vi "Set Velocity Setpoint.vi"(8 "error in (no error)":errorcluster, 10 "CCW Velocity (0 rad/s)":dbl, 11 "DC Motor Controller in":refnum<class "DC Motor Controller.lvclass">) -> (0 "error out":errorcluster, 3 "DC Motor Controller out":refnum<class "DC Motor Controller.lvclass">)   [LabVIEW 2019, in "DC Motor Controller.lvclass"]
doc: "Sets the counterclockwise velocity setpoint of the motor."
uses:
  DC Motor Controller.lvclass
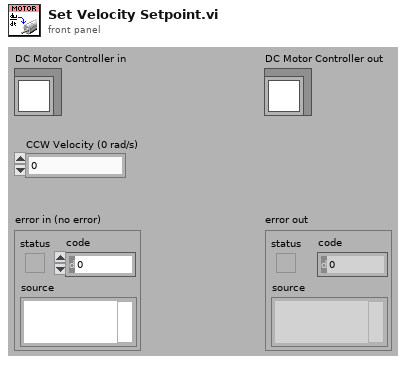
[diagram p1: front panel]
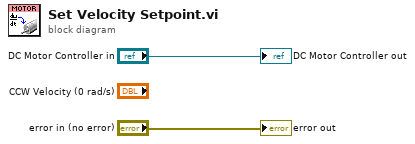
[diagram p0: block diagram]
diagram:
  "error out" <- "error in (no error)"
  "DC Motor Controller out" <- "DC Motor Controller in"
